vi "CF-check_file_path.vi"(10 "File Path":path) -> (2 "File Path out":path)   [LabVIEW 2020, in "CF-common_features.lvlib"]
uses:
  CF-common_features.lvlib
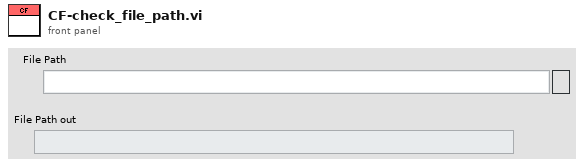
[diagram p1: front panel]
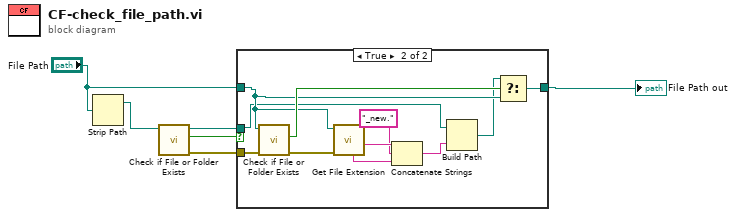
[diagram p0: block diagram]
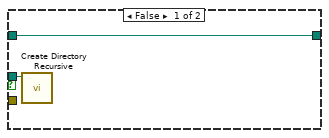
[diagram p2: hidden frame]
diagram:
  n1 = Strip Path(path="File Path") -> (stripped path=w6:path)  [unwired: 1 out]
  n2 = call <vilib>:"Check if File or Folder Exists.vi"("path"=w6) -> ("error out"=w1:errorcluster, "file or folder exists?"=w5:bool, "dup path"=w4:path)  [unwired: 8 in]
  n3 = case shown="True" w5 {
    tunnel: w4 -> [w8 w10]
    tunnel: "File Path" -> [w7 w12]
    tunnel: [w7 w18] -> w2
    tunnel: w1 -> [_ w17]
    frame False {
      n4 = call <vilib>:"Create Directory Recursive.vi"("directory"=w8) -> ()  [unwired: 4 in, 3 out]
    }
    frame True {
      n5 = call <vilib>:"Check if File or Folder Exists.vi"("error in (no error)"=w17, "path"=w12) -> ("error out"=w16:errorcluster, "file or folder exists?"=w19:bool)  [unwired: 7 in, 1 out]
      n6 = call <vilib>:"Get File Extension.vi"("error in (no error)"=w16, "file"=w12) -> ("filename without extension"=w15:string, "unmodified file extension"=w13:string)  [unwired: 5 in, 3 out]
      n7 = Concatenate Strings(w15, "_new." ("string"), w13) -> (w11:string)
      n8 = Build Path(base path=w10, name or relative path=w11) -> (appended path=w9:path)
      n9 = Select(t=w9, s=w19, f=w12) -> (s? t:f=w18:path)
    }
  }
  "File Path out" <- w2
